vi "3_Generate_pulse_on_one_channel.vi"() -> ()   [LabVIEW 2014]
uses:
  <vilib>/Swabian Instruments/Pulse Streamer/PulseStreamer/PulseStreamer/typedefs/typedef_TriggerStart.ctl
  <vilib>/Swabian Instruments/Pulse Streamer/PulseStreamer/PulsePattern/PulsePattern.lvclass
  <vilib>/Swabian Instruments/Pulse Streamer/PulseStreamer/typedefs/typedef_ChannelNumber.ctl
  <vilib>/Swabian Instruments/Pulse Streamer/PulseStreamer/Sequence/Sequence.lvclass
  <vilib>/Swabian Instruments/Pulse Streamer/PulseStreamer/PulseStreamer/stream/stream (Sequence).vi
  <vilib>/Swabian Instruments/Pulse Streamer/PulseStreamer/PulseStreamer/PulseStreamer.lvclass
  <vilib>/Swabian Instruments/Pulse Streamer/PulseStreamer/PulseStreamer.lvlib
panel:
  in  "ip or hostname":string="pulsestreamer"
  in  "Level 3":bool
  in  "Duration 3":u64=1000
  out "error out":errorcluster
  in  "nRuns":i64=-1
  in  "Start Type":T1
  in  "Duration 2":u64=500
  in  "Duration 1":u64=1000
  in  "Level 2":bool=TRUE
  in  "Level 1":bool
  # "This example demonstrates how to generate simple square pulse on output channel \"0\" \nThe pulse can be repeated finite or infinite number of times by specifying value of \"nRuns\"."
  # "'nRuns' defines how many time the sequence has to be repeated by hardware\nnRuns<0 means that sequence will be repeated indefinitely"
  # "Defines whether the sequence starts \n* immediatly after it was uploaded  (IMMEDIATE)\n* after a software trigger (startNow) has been sent (SOFTWARE)\n* with an external trigger signal to \"Trigger\" input on the corresponding edge (HW_RISING, HW_FALLING, HW_BOTH)."
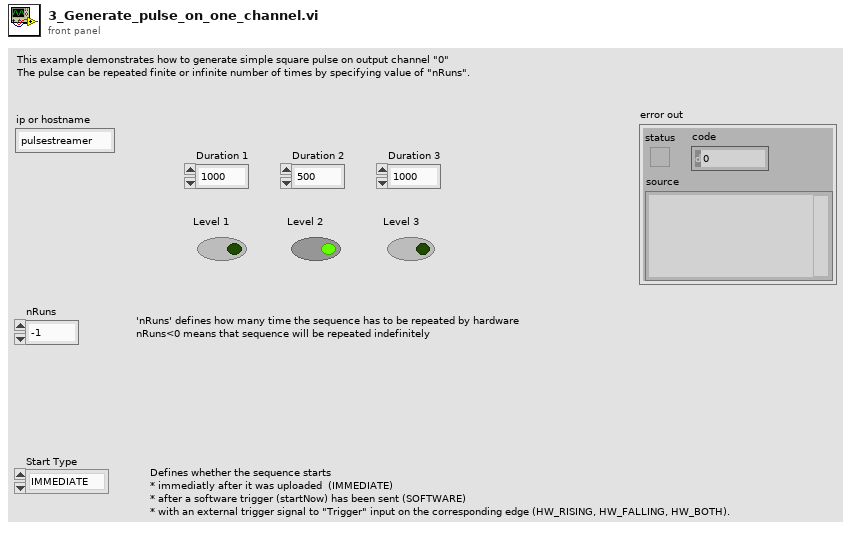
[diagram p1: front panel]
types:
  T1 = typedef "PulseStreamer.lvlib/PulseStreamer.lvclass/typedef_TriggerStart.ctl" = enum16{"IMMEDIATE", "SOFTWARE", "HW_RISING", "HW_FALLING", "HW_RISING_AND_FALLING"}
  T2 = typedef "PulseStreamer.lvlib/typedef_ChannelNumber.ctl" = i16
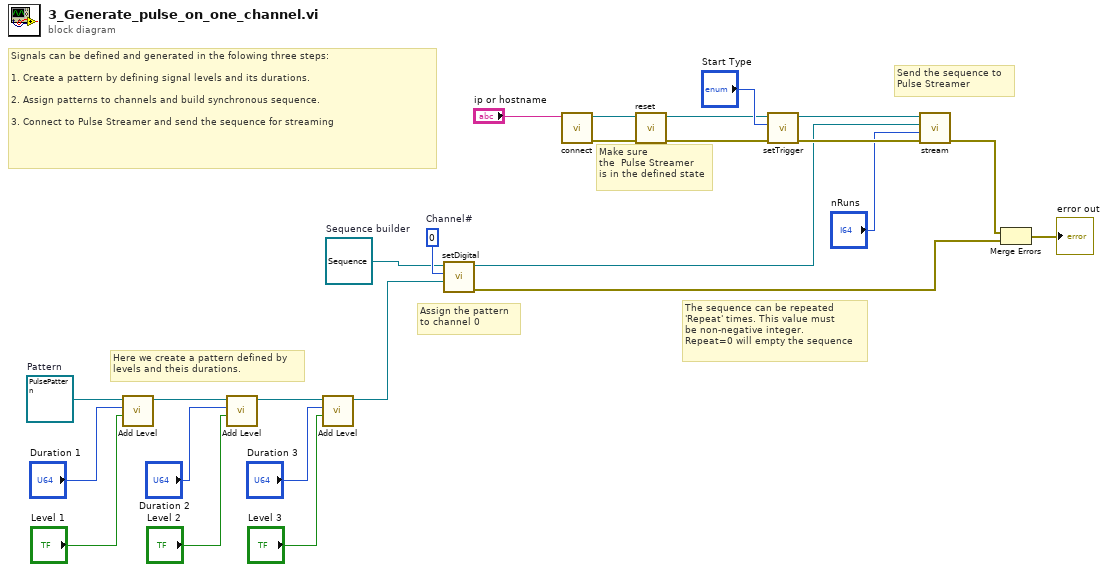
[diagram p0: block diagram]
diagram:
  w13 = refnum<class "Sequence.lvclass"> refnum  # Sequence builder
  w18 = T2 0  # Channel#
  w23 = refnum<class "PulsePattern.lvclass"> refnum  # Pattern
  # "Make sure\nthe  Pulse Streamer\nis in the defined state"
  # "Send the sequence to \nPulse Streamer"
  # "The sequence can be repeated\n'Repeat' times. This value must \nbe non-negative integer.\nRepeat=0 will empty the sequence"
  # "Assign the pattern \nto channel 0"
  # "Here we create a pattern defined by \nlevels and theis durations."
  # "Signals can be defined and generated in the folowing three steps:\n\n1. Create a pattern by defining signal levels and its durations.\n\n2. Assign patterns to channels and build synchronous sequence.\n\n3. Connect to Pulse Streamer and send the sequence for streaming"
  n1 = call <vilib>:"Add Level.vi"("Level"="Level 1", "Duration"="Duration 1", "Digital Sequence in"=w23) -> ("Digital Sequence out"=w25:refnum<class "PulsePattern.lvclass">)  [unwired: 8 in]
  n2 = call <vilib>:"Add Level.vi"("Level"="Level 2", "Duration"="Duration 2", "Digital Sequence in"=w25) -> ("Digital Sequence out"=w24:refnum<class "PulsePattern.lvclass">)  [unwired: 8 in]
  n3 = call <vilib>:"Add Level.vi"("Level"="Level 3", "Duration"="Duration 3", "Digital Sequence in"=w24) -> ("Digital Sequence out"=w16:refnum<class "PulsePattern.lvclass">)  [unwired: 8 in]
  n4 = call-dynamic "setDigital.vi"("PulsePattern"=w16, "channel"=w18, "Sequence in"=w13) -> ("error out"=w17:errorcluster, "Sequence out"=w1:refnum<class "Sequence.lvclass">)  [unwired: 7 in]
  n5 = call <vilib>:"connect.vi"("ip"="ip or hostname") -> ("error out"=w10:errorcluster, "Pulse Streamer out"=w12:refnum<class "PulseStreamer.lvclass">)  [unwired: 9 in]
  n6 = call <vilib>:"reset.vi"("error in (no error)"=w10, "Pulse Streamer in"=w12) -> ("error out"=w9:errorcluster, "Pulse Streamer out"=w11:refnum<class "PulseStreamer.lvclass">)  [unwired: 8 in]
  n7 = call-dynamic "setTrigger.vi"("error in (no error)"=w9, "start"="Start Type", "Pulse Streamer in"=w11) -> ("error out"=w21:errorcluster, "Pulse Streamer out"=w22:refnum<class "PulseStreamer.lvclass">)  [unwired: 7 in]
  n8 = call-poly <vilib>:"stream.vi"("error in (no error)"=w21, "n_runs"="nRuns", "sequence"=w1, "Pulse Streamer in"=w22) -> ("error out"=w14:errorcluster)  [unwired: 4 in, 1 out]
  n9 = Merge Errors(w14, w17) -> (→"error out":errorcluster)
